vi "ReadXML2.vi"(7 "ParamsUI 2":T1={"IsNorImage"=FALSE, "Exposure Values"=0, "ImagePath"=path "", "Inspection Number"=3}, 10 "Name":string="A1", 11 "基路径":path) -> (3 "ParamsUI 3":T1={"IsNorImage"=FALSE, "Exposure Values"=0, "ImagePath"=path "", "Inspection Number"=3})   [LabVIEW 2015]
uses:
  <vilib>/Utility/xml.llb/Read From XML File(string).vi
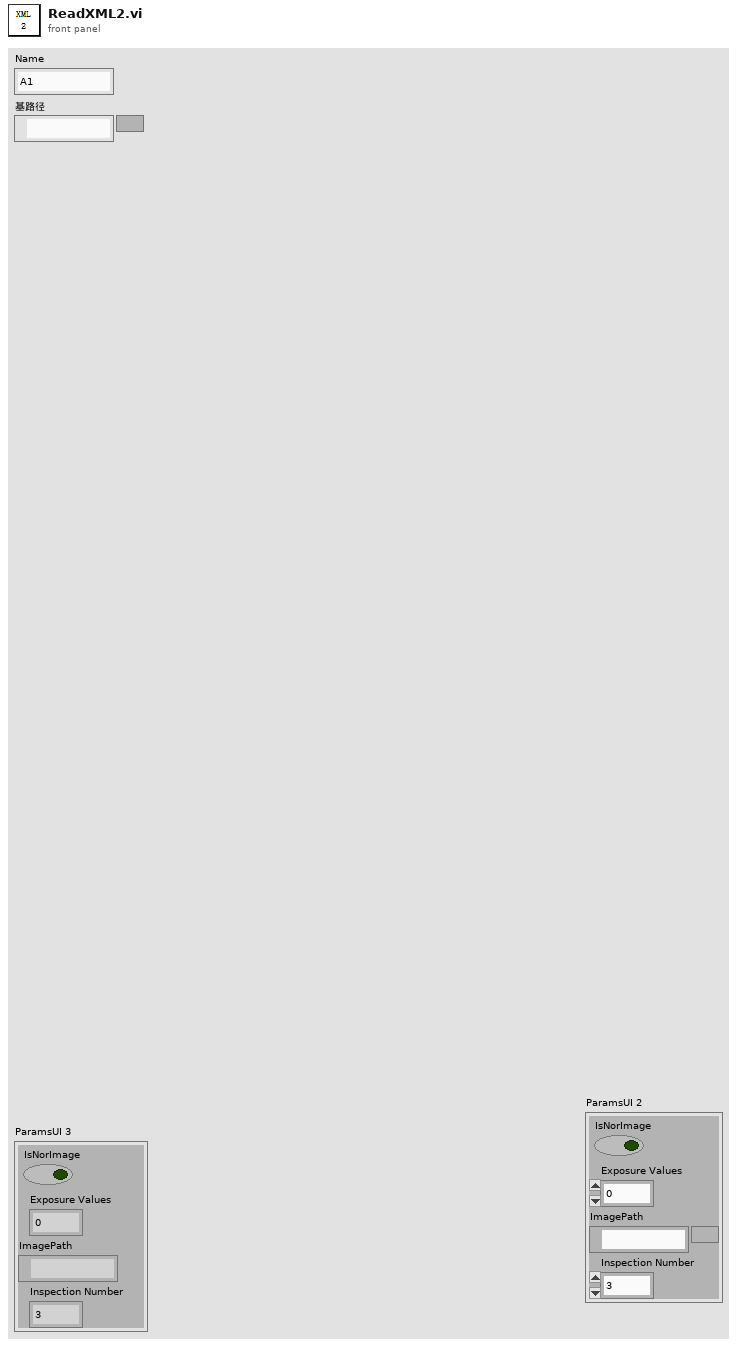
[diagram p1: front panel]
types:
  T1 = cluster{"IsNorImage":bool, "Exposure Values":u32, "ImagePath":path, "Inspection Number":i32}
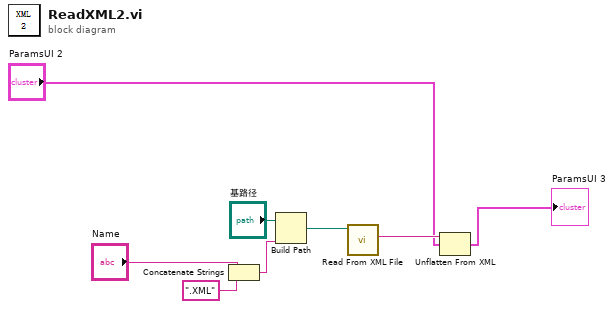
[diagram p0: block diagram]
diagram:
  n1 = Concatenate Strings("Name", ".XML" ("字符串")) -> (w4:string)
  n2 = Build Path(base path="基路径", name or relative path=w4) -> (appended path=w8:path)
  n3 = call-poly <vilib>:"Read From XML File.vi"("XML File Path"=w8) -> ("XML Elements"=w7:string)  [unwired: 8 in, 2 out]
  n4 = Unflatten From XML(xml string=w7, type="ParamsUI 2") -> (value=→"ParamsUI 3":T1)  [unwired: 1 in, 1 out]
